vi "Headers & Data String to File v2.vi"(4 "Header String":string, 5 "Data Line String":string, 6 "error in (no error)":errorcluster, 7 "pos mode (rel. to end:1)":enum16{"start", "end", "current"}(ring)=enum."end", 8 "operation":T1(ring)=enum."open or create", 9 "File Path":path=path "C:/ssdata.txt") -> (0 "error out":errorcluster, 3 "Path Out":path)   [LabVIEW 2020]
doc: "This vi is intended to write an externally formatted (usually using Array to Ssht String) data line string to a delimited text file with column headers that can be imported to Excel or other analysis programs. \n\nThe file is opened then closed each time it is written to, which is good for lower speed (seconds per sample, vs. samples per second) data acquisition. The headers are only written when the file is first opened and Open/Create/Replace File.vi reports its size to be zero. Several rows of headers can be supplied as a 2d string array. This string inputcan be anything, but check your analysis application to see what it will accept. MS apps such as Excel will accept and display many formats, but convert time internally to a floating point value in Days Since 1/1/1900, 00:00:00). \n-W.J. Gilbert, 4/2/2002"
panel:
  in  "format string":string="%s"
  # "Header String is only written once, when the file is newly opened, and file size is zero.. Time string is eternally formatted, and is prepended to each data line separated by delimiter character."
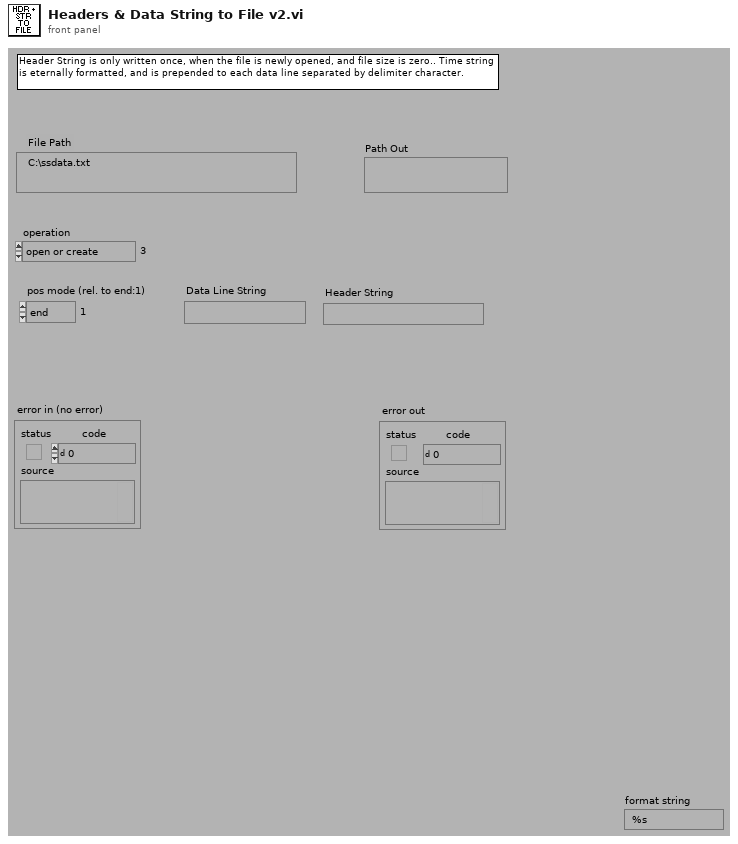
[diagram p1: front panel]
types:
  T1 = enum16{"open", "replace", "create", "open or create", "replace or create", "replace or create with confirmation"}
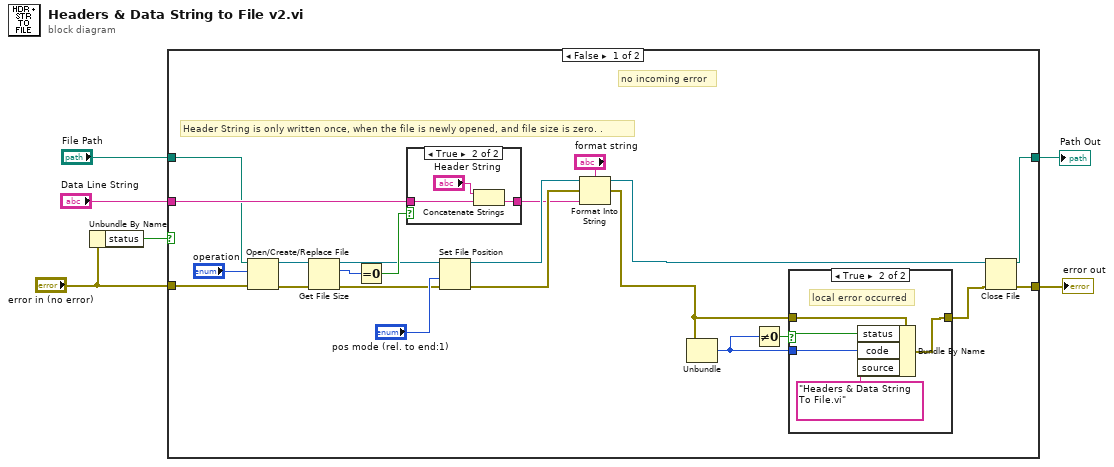
[diagram p0: block diagram]
diagram:
  n1 = Unbundle By Name("error in (no error)") -> ("status"=w6:bool)
  n2 = case shown="False" w6 {
    tunnel: [w28 w40] -> w4
    tunnel: "error in (no error)" -> [w22 w40]
    tunnel: "Data Line String" -> [w26 _]
    tunnel: "File Path" -> [w10 w39]
    tunnel: [w9 w39] -> w1
    frame False {
      # "no incoming error"
      # "Header String is only written once, when the file is newly opened, and file size is zero. ."
      n3 = Open/Create/Replace File(file path (use dialog)=w10, error in=w22, operation (0:open)="operation") -> (refnum out=w23:refnum<file>, error out=w24:errorcluster)  [unwired: 3 in, 1 out]
      n4 = Get File Size(file=w23, error in=w24) -> (refnum out=w13:refnum<file>, size (in bytes)=w21:i64, 0:w14:errorcluster)
      n5 = Equal To 0?(x=w21) -> (x = 0?=w27:bool)
      n6 = case shown="True" w27 {
        tunnel: w26 -> [w35 w37]
        tunnel: [w35 w36] -> w12
        frame False {
        }
        frame True {
          n7 = Concatenate Strings("Header String", w37) -> (w36:string)
        }
      }
      n8 = Set File Position(refnum=w13, from (0:start)="pos mode (rel. to end:1)", error in=w14) -> (refnum out=w18:refnum<file>, error out=w17:errorcluster)  [unwired: 1 in]
      n9 = Format Into String(format string="format string", initial string=w18, error in=w17, w12) -> (resulting string=w8:refnum<file>, error out=w7:errorcluster)
      n10 = Unbundle(w7) -> ("code"=w19:i32)  [unwired: 2 out]
      n11 = Not Equal To 0?(x=w19) -> (x != 0?=w20:bool)
      n12 = case shown="True" w20 {
        selector: w20 -> [_ w31]
        tunnel: w19 -> [_ w33]
        tunnel: [w29 w32] -> w11
        tunnel: w7 -> [w29 w30]
        frame False {
          # "no local error"
        }
        frame True {
          # "local error occurred"
          n13 = Bundle By Name(cluster=w30, "status"=w31, "code"=w33, "source"="Headers & Data String To File.vi") -> (w32:errorcluster)
        }
      }
      n14 = Close File(refnum=w8, error in=w11) -> (path=w9:path, error out=w28:errorcluster)
    }
    frame True {
    }
  }
  "error out" <- w4
  "Path Out" <- w1
